vi "TrajectoryConfig_GetVoltageDiffDriveConstraint.vi"(11 "inTRAJECTORY_CONFIG":T1 {"End Velocity" format="%20.4f"; "StartVelocity" format="%20.4f"; "Max Acceleration" format="%20.4f"; "MaxVelocity" format="%20.4f"}) -> (1 "Constraint Exists":bool, 3 "Differential Drive Voltage Constraint":T2 {"SIMPLE_MOTOR_FF"."KnInv" format="%13.4f"; "SIMPLE_MOTOR_FF"."Ka" format="%13.4f"; "SIMPLE_MOTOR_FF"."Kv" format="%13.4f"; "SIMPLE_MOTOR_FF"."Ks" format="%13.4f"; "DIFF_DRIVE_KINEMATICS"."TrackWidth_Meters" format="%20.4f"; "Max Voltage" format="%20.4f"})   [LabVIEW 2019, in "Trajectory_Library.lvlib"]
doc: "Retrieves the Differential Drive voltage constraint from the Trajectory Configuration.\n\nNote: If more than once instance of the Differential Drive Voltage constraint exists only the first one is returned. (Only one of these should be defined.)\n\nParameters:\n - InTrajectoryConfig -- The trajectory configuration data structure\n\nReturns:\n - Diff Drive Voltage Constraint -- The data cluster containing the constraint.\n - Constraint Exists -- Returns TRUE if this constraint is defined in the trjaectory configuration."
uses:
  Trajectory_Library.lvlib
  <vilib>/Utility/Data Type/NI_Data Type.lvlib
  TypeDef/DIFF_DRIVE_KINEMATICS.ctl
  TypeDef/SIMPLE_MOTOR_FF.ctl
  TypeDef/TRAJ_CONSTRAINT_DIIF_DRIVE_VOLTAGE.ctl
  TypeDef/TRAJ_CONFIG.ctl
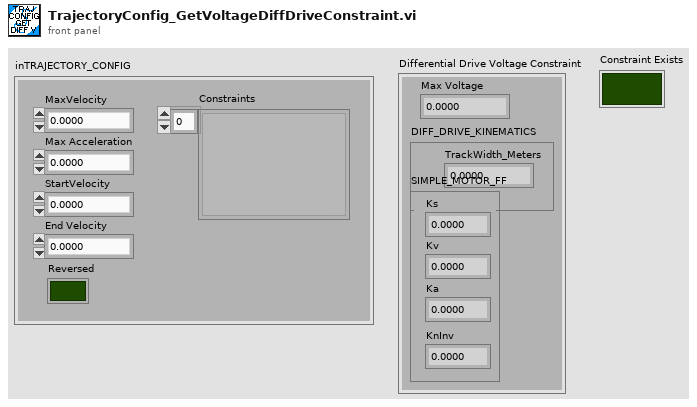
[diagram p1: front panel]
types:
  T1 = typedef "Trajectory_Library.lvlib/TRAJ_CONFIG.ctl" = cluster{"MaxVelocity":dbl, "Max Acceleration":dbl, "StartVelocity":dbl, "End Velocity":dbl, "Reversed":bool, "Constraints":variant[]}
  T2 = typedef "Trajectory_Library.lvlib/TRAJ_CONSTRAINT_DIIF_DRIVE_VOLTAGE.ctl" = cluster{"Max Voltage":dbl, "DIFF_DRIVE_KINEMATICS":T3, "SIMPLE_MOTOR_FF":T4}
  T3 = typedef "Trajectory_Library.lvlib/DIFF_DRIVE_KINEMATICS.ctl" = cluster{"TrackWidth_Meters":dbl}
  T4 = typedef "Trajectory_Library.lvlib/SIMPLE_MOTOR_FF.ctl" = cluster{"Ks":dbl, "Kv":dbl, "Ka":dbl, "KnInv":dbl}
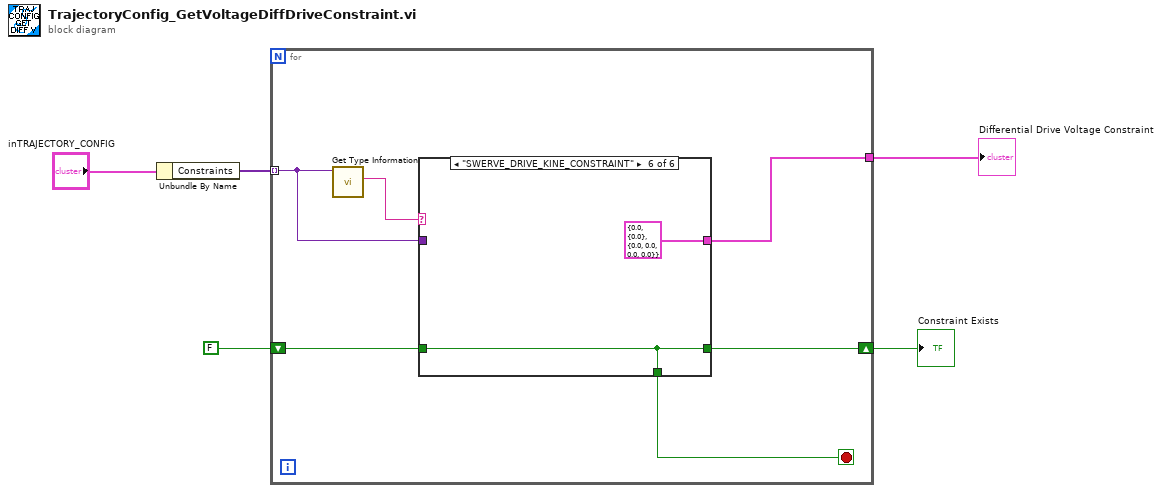
[diagram p0: block diagram]
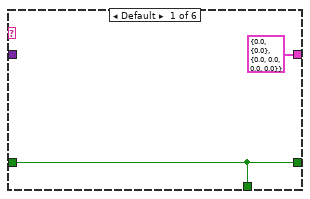
[diagram p2: hidden frame]
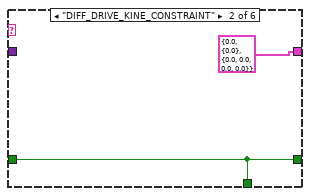
[diagram p3: hidden frame]
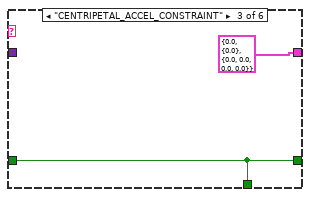
[diagram p4: hidden frame]
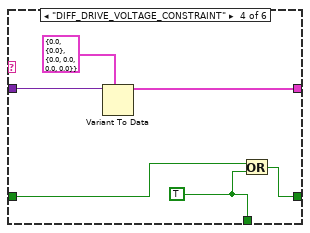
[diagram p5: hidden frame]
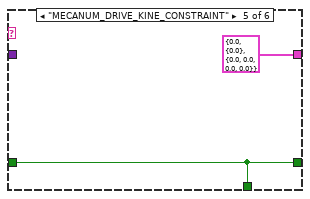
[diagram p6: hidden frame]
diagram:
  n1 = Unbundle By Name("inTRAJECTORY_CONFIG") -> ("Constraints"=w2:variant[])
  n2 = for {
    tunnel: w2 -> [w10] mode=indexing
    shift-right: [w8] -> w4
    shift-left: FALSE -> [w9]
    tunnel: [w6] -> w1
    stop <- w7 stop-if-true
    n3 = call <vilib>:"Get Type Information.vi"("variant"=w10) -> ("name"=w11:string)  [unwired: 6 in, 4 out]
    n4 = case shown="\"SWERVE_DRIVE_KINE_CONSTRAINT\"" w11 {
      tunnel: w10 -> [_ _ _ w22 _ _]
      tunnel: w9 -> [w12 w15 w16 w19 w24 w27]
      tunnel: [w12 w15 w16 w20 w24 w27] -> w8
      tunnel: [w12 w15 w16 w18 w24 w27] -> w7
      tunnel: [T2 {"Max Voltage"=0.0, "DIFF_DRIVE_KINEMATICS"={"TrackWidth_Meters"=0.0}, "SIMPLE_MOTOR_FF"={"Ks"=0.0, "Kv"=0.0, "Ka"=0.0, "KnInv"=0.0}} ("DIFF_DRIVE_VOLTAGE_CONSTRAINT") T2 {"Max Voltage"=0.0, "DIFF_DRIVE_KINEMATICS"={"TrackWidth_Meters"=0.0}, "SIMPLE_MOTOR_FF"={"Ks"=0.0, "Kv"=0.0, "Ka"=0.0, "KnInv"=0.0}} ("DIFF_DRIVE_VOLTAGE_CONSTRAINT") T2 {"Max Voltage"=0.0, "DIFF_DRIVE_KINEMATICS"={"TrackWidth_Meters"=0.0}, "SIMPLE_MOTOR_FF"={"Ks"=0.0, "Kv"=0.0, "Ka"=0.0, "KnInv"=0.0}} ("DIFF_DRIVE_VOLTAGE_CONSTRAINT") w21 T2 {"Max Voltage"=0.0, "DIFF_DRIVE_KINEMATICS"={"TrackWidth_Meters"=0.0}, "SIMPLE_MOTOR_FF"={"Ks"=0.0, "Kv"=0.0, "Ka"=0.0, "KnInv"=0.0}} ("DIFF_DRIVE_VOLTAGE_CONSTRAINT") T2 {"Max Voltage"=0.0, "DIFF_DRIVE_KINEMATICS"={"TrackWidth_Meters"=0.0}, "SIMPLE_MOTOR_FF"={"Ks"=0.0, "Kv"=0.0, "Ka"=0.0, "KnInv"=0.0}} ("DIFF_DRIVE_VOLTAGE_CONSTRAINT")] -> w6
      frame Default {
      }
      frame "DIFF_DRIVE_KINE_CONSTRAINT" {
      }
      frame "CENTRIPETAL_ACCEL_CONSTRAINT" {
      }
      frame "DIFF_DRIVE_VOLTAGE_CONSTRAINT" {
        w18 = TRUE
        n5 = Variant To Data(type=T2 {"Max Voltage"=0.0, "DIFF_DRIVE_KINEMATICS"={"TrackWidth_Meters"=0.0}, "SIMPLE_MOTOR_FF"={"Ks"=0.0, "Kv"=0.0, "Ka"=0.0, "KnInv"=0.0}} ("DIFF_DRIVE_VOLTAGE_CONSTRAINT"), Variant=w22) -> (data=w21:T2)  [unwired: 1 in, 1 out]
        n6 = Or(x=w19, y=w18) -> (x .or. y?=w20:bool)
      }
      frame "MECANUM_DRIVE_KINE_CONSTRAINT" {
      }
      frame "SWERVE_DRIVE_KINE_CONSTRAINT" {
      }
    }
  }
  "Differential Drive Voltage Constraint" <- w1
  "Constraint Exists" <- w4
